vi "Date Setup.vi"(0 "VISA resource name":refnum<visa-resource-name>, 1 "Hour":i16=1 min=1 max=31, 2 "Minute":i16=1 min=1 max=31, 3 "Second":i16=1 min=1 max=31, 5 "Date":i16=31 min=1 max=31, 7 "Month":i16=12 min=1 max=12, 9 "Year":i16=2001 min=2000 max=2099, 11 "error in (no error)":errorcluster) -> (4 "VISA resource name out":refnum<visa-resource-name>, 15 "error out":errorcluster)   [LabVIEW 2021, in "Siglent SDS 1000 2000 Series.lvlib"]
doc: "Sets up date and time in the CFL series instrument."
uses:
  <instrlib>/Siglent SDS 1000 2000 Series/Siglent SDS 1000 2000 Series.lvlib
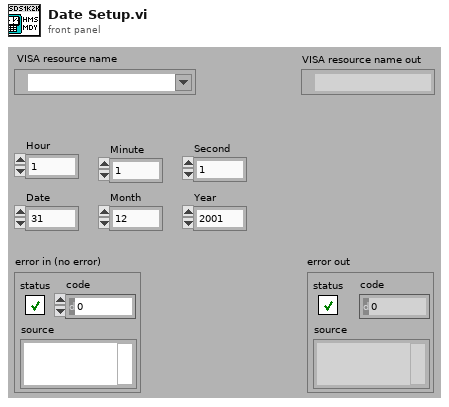
[diagram p1: front panel]
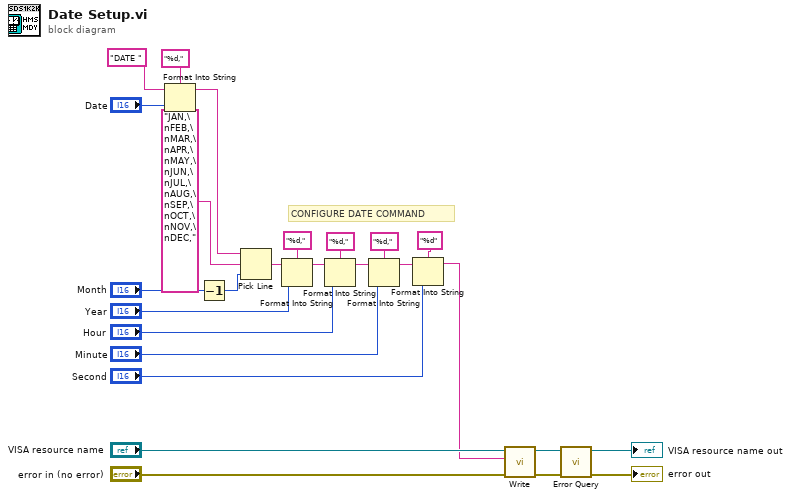
[diagram p0: block diagram]
diagram:
  # "CONFIGURE DATE COMMAND"
  n1 = Format Into String(format string="%d,", initial string="DATE ", "Date") -> (resulting string=w18:string)  [unwired: 1 in, 1 out]
  n2 = Decrement(x="Month") -> (x-1=w23:i16)
  n3 = Pick Line(string ("")=w18, multi-line string="JAN,\nFEB,\nMAR,\nAPR,\nMAY,\nJUN,\nJUL,\nAUG,\nSEP,\nOCT,\nNOV,\nDEC,", line index=w23) -> (output string=w17:string)
  n4 = Format Into String(format string="%d,", initial string=w17, "Year") -> (resulting string=w13:string)  [unwired: 1 in, 1 out]
  n5 = Format Into String(format string="%d,", initial string=w13, "Hour") -> (resulting string=w10:string)  [unwired: 1 in, 1 out]
  n6 = Format Into String(format string="%d,", initial string=w10, "Minute") -> (resulting string=w6:string)  [unwired: 1 in, 1 out]
  n7 = Format Into String(format string="%d", initial string=w6, "Second") -> (resulting string=w5:string)  [unwired: 1 in, 1 out]
  n8 = call <instrlib>:"Write.vi"("error in (no error)"="error in (no error)", "Write Buffer"=w5, "VISA resource name"="VISA resource name") -> ("error out"=w4:errorcluster, "VISA resource name out"=w3:refnum<visa-resource-name>)  [unwired: 6 in, 1 out]
  n9 = call <instrlib>:"Error Query.vi"("error in (no error)"=w4, "VISA resource name"=w3) -> ("error out"=→"error out":errorcluster, "VISA resource name out"=→"VISA resource name out":refnum<visa-resource-name>)  [unwired: 6 in, 2 out]
